vi "MB Ethernet Wait on Query.vi"(9 "Data Reference":T1, 10 "Timeout":i32=25000, 11 "Connection ID":refnum<k5>) -> ()   [LabVIEW 2019, in "NI_modbus_upd.lvlib"]
uses:
  NI_modbus_upd.lvlib
  Ctl/MB Ethernet Connection Function.ctl
  MB Globals.vi
panel:
  # "VI Name: MB Ethernet Wait on Query.vi\nPurpose: Serves a Modbus TCP query.\nReentrant VI called dynamically, so that multiple\nqueries can be served in parallel."
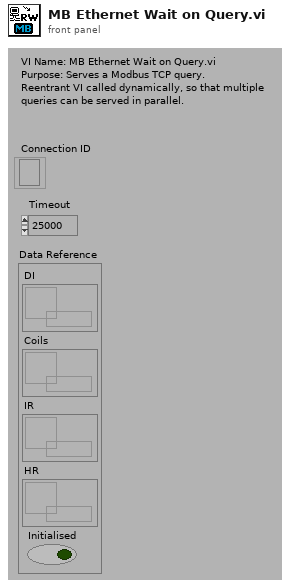
[diagram p1: front panel]
types:
  T1 = cluster{"DI":refnum<data-value>, "Coils":refnum<data-value>, "IR":refnum<data-value>, "HR":refnum<data-value>, "Initialised":bool}
  T2 = typedef "NI_modbus_upd.lvlib/MB Ethernet Connection Function.ctl" = enum16{"Init", "Add Connection", "Get All Connections", "Delete Connection"}
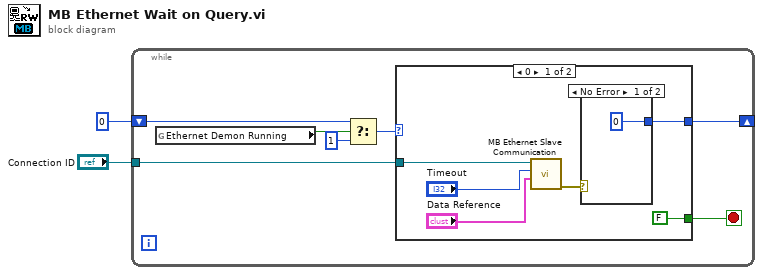
[diagram p0: block diagram]
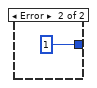
[diagram p2: hidden frame]
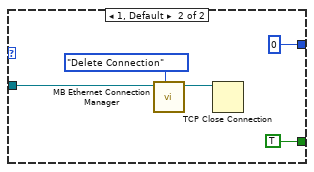
[diagram p3: hidden frame]
diagram:
  n1 = while {
    shift-right: [w9] -> _
    shift-left: 0 -> [w5]
    tunnel: "Connection ID" -> [w7]
    stop <- w8 stop-if-true
    n2 = global read "MB Globals.vi" "Ethernet Demon Running"() -> (w6:bool)
    n3 = Select(t=w5, s=w6, f=1) -> (s? t:f=w3:i32)
    n4 = case shown="0" w3 {
      tunnel: w7 -> [w15 w18]
      tunnel: [w12 0] -> w9
      tunnel: [FALSE TRUE] -> w8
      frame 0 {
        n5 = call "MB Ethernet Slave Communication.vi"("Data Reference"="Data Reference", "Timeout"="Timeout", "Connection ID"=w15) -> ("error out"=w14:errorcluster)  [unwired: 7 in, 1 out]
        n6 = case shown="No Error" w14 {
          tunnel: [0 1] -> w12
          frame No Error {
          }
          frame Error {
          }
        }
      }
      frame 1, Default {
        n7 = call "MB Ethernet Connection Manager.vi"("Function"=MB_Ethernet_Connection_Function."Delete Connection", "Connection ID"=w18) -> ("Connection ID to Delete"=w19:refnum<k5>)  [unwired: 7 in, 2 out]
        n8 = TCP Close Connection(connection ID=w19) -> ()  [unwired: 2 in, 2 out]
      }
    }
  }
